vi "Analog FGlobal.vi"(0 "System no.":i32=1 min=1 step=1, 1 "Read(F)/Write":bool=TRUE, 2 "VI ref in":refnum<vi>) -> (16 "VI ref out":refnum<vi>)   [LabVIEW 2020]
doc: "This VI works as a functional global variable for VI references\n\nValid for Analog Systems, but must be present for all other systems, too."
panel:
  out "VI ref":refnum<vi>[](array[refnum])
  # "This VI works as a functional global variable for VI references."
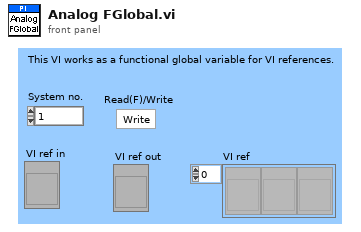
[diagram p1: front panel]
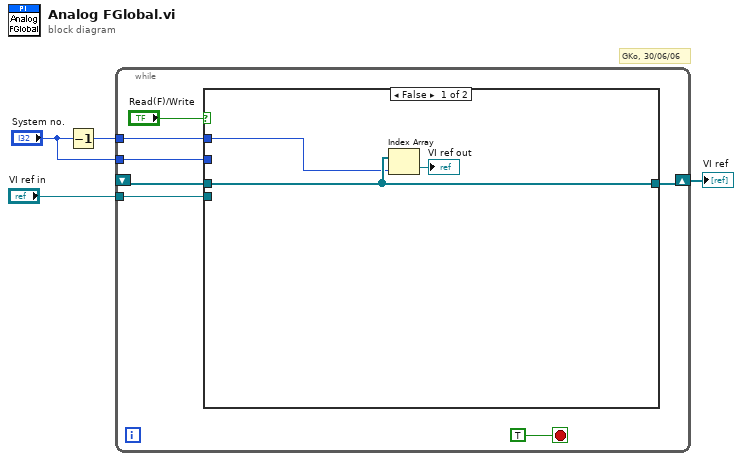
[diagram p0: block diagram]
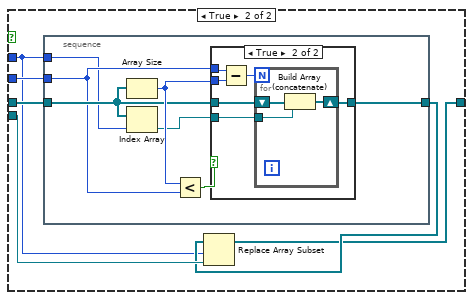
[diagram p2: hidden frame]
diagram:
  # "GKo, 30/06/06"
  n1 = Decrement(x="System no.") -> (x-1=w4:i32)
  n2 = while {
    shift-right: [w8] -> w1
    shift-left: _ -> [w9]
    tunnel: w4 -> [w7]
    tunnel: "System no." -> [w6]
    tunnel: "VI ref in" -> [w5]
    stop <- TRUE stop-if-true
    n3 = case shown="False" "Read(F)/Write" {
      tunnel: w9 -> [w14 w20]
      tunnel: [w14 w16] -> w8
      tunnel: w7 -> [w12 w15]
      tunnel: w6 -> [_ w19]
      tunnel: w5 -> [_ w18]
      frame False {
        n4 = Index Array(array=w14, index=w12) -> (element=→"VI ref out":refnum<vi>)
      }
      frame True {
        n5 = stacked-sequence {
          tunnel: w20 -> [w24]
          tunnel: [w23] -> w17
          tunnel: w15 -> [w21]
          tunnel: w19 -> [w22]
          frame #0 {
            n6 = Array Size(array=w24) -> (size(s)=w26:i32)
            n7 = Index Array(array=w24, index=w21) -> (element=w25:refnum<vi>)
            n8 = Less?(x=w26, y=w22) -> (x < y?=w27:bool)
            n9 = case shown="True" w27 {
              tunnel: w22 -> [_ w33]
              tunnel: w26 -> [_ w32]
              tunnel: w24 -> [w28 w31]
              tunnel: w25 -> [_ w30]
              tunnel: [w28 w29] -> w23
              frame False {
              }
              frame True {
                n10 = Subtract(x=w33, y=w32) -> (x-y=w34:i32)
                n11 = for {
                  N: w34 -> [_]
                  shift-right: [w37] -> w29
                  shift-left: w31 -> [w36]
                  tunnel: w30 -> [w35]
                  n12 = Build Array (concatenate)(w36, w35) -> (w37:refnum<vi>[])
                }
              }
            }
          }
        }
        n13 = Replace Array Subset(array=w17, new element=w18, index=w15) -> (w16:refnum<vi>[])
      }
    }
  }
  "VI ref" <- w1
